vi "Ramsete_Execute_PackTuning_ENG.vi"(5 "B":dbl=2.0, 6 "Heading Tolerance DEG":dbl=0.035, 7 "Zeta":dbl=0.7, 8 "Y Tolerance Ft":dbl=0.051, 9 "X Tolerance Ft":dbl=0.051, 10 "Max Speed Ft/S":dbl, 11 "Track Width Ft":dbl) -> (3 "RAMSETE_EXE_TUNING":T1={"B"=2.0, "Zeta"=0.7, "X Tolerance M"=2.0, "Y Tolerance M"=0.7, "Heading Tolerance RAD"=0.7, "Track Width M"=2.0, "Max Speed M/S"=2.0} {"Max Speed M/S" format="%13.4f"; "Track Width M" format="%13.4f"; "Heading Tolerance RAD" format="%13.4f"; "Y Tolerance M" format="%13.4f"; "X Tolerance M" format="%13.4f"; "Zeta" format="%13.4f"; "B" format="%13.4f"})   [LabVIEW 2019, in "Trajectory_Library.lvlib"]
doc: "Packs tuning parameters for the Ramsete EXE VI (Which is designed for a differential drive robot)\n\nThis verion uses ENG input units (Ft, Degs)"
uses:
  RAMSETE_EXE_TUNING.ctl
  Trajectory_Library.lvlib
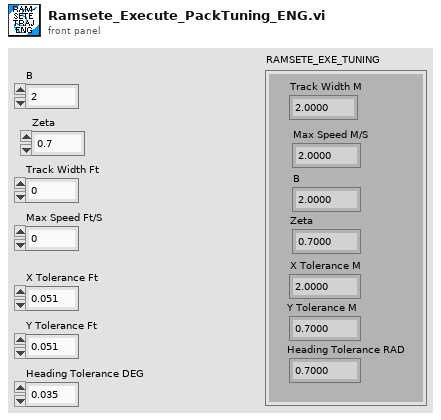
[diagram p1: front panel]
types:
  T1 = typedef "Trajectory_Library.lvlib/RAMSETE_EXE_TUNING.ctl" = cluster{"B":dbl, "Zeta":dbl, "X Tolerance M":dbl, "Y Tolerance M":dbl, "Heading Tolerance RAD":dbl, "Track Width M":dbl, "Max Speed M/S":dbl}
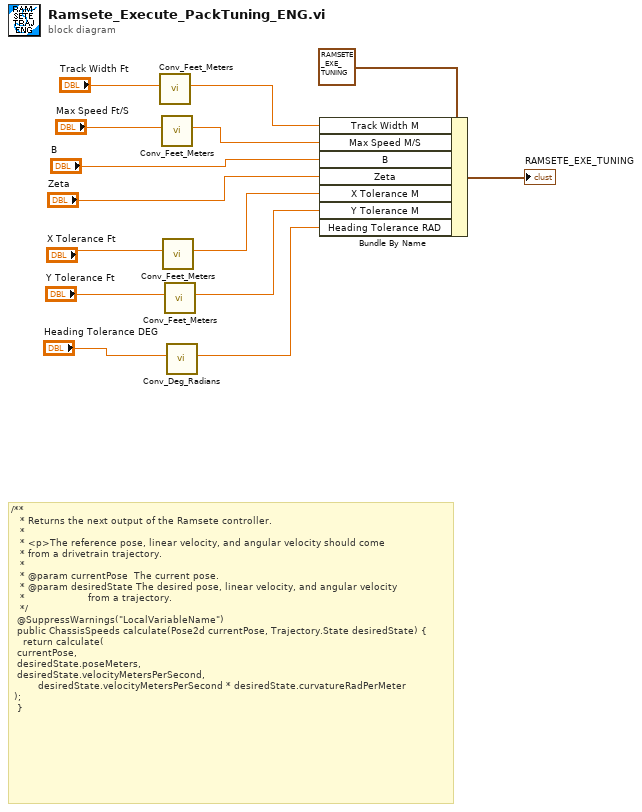
[diagram p0: block diagram]
diagram:
  # "/**\n   * Returns the next output of the Ramsete controller.\n   *\n   * <p>The reference pose, linear velocity, and angular velocity should come\n   * from a drivetrain trajectory.\n   *\n   * @param currentPose  The current pose.\n   * @param desiredState The desired pose, linear velocity, and angular velocity\n   *                     from a trajectory.\n   */\n  @SuppressWarnings(\"LocalVariableName\")\n  public ChassisSpeeds calculate(Pose2d currentPose, Trajectory.State desiredState) {\n    return calculate(\n\t\tcurrentPose, \n\t\tdesiredState.poseMeters, \n\t\tdesiredState.velocityMetersPerSecond,\n        \tdesiredState.velocityMetersPerSecond * desiredState.curvatureRadPerMeter\n\t);\n  }"
  n1 = call "Conv_Feet_Meters.vi"("Feet"="Track Width Ft") -> ("Meters"=w1:dbl)  [unwired: 10 in]
  n2 = call "Conv_Feet_Meters.vi"("Feet"="Max Speed Ft/S") -> ("Meters"=w4:dbl)  [unwired: 10 in]
  n3 = call "Conv_Feet_Meters.vi"("Feet"="X Tolerance Ft") -> ("Meters"=w6:dbl)  [unwired: 10 in]
  n4 = call "Conv_Feet_Meters.vi"("Feet"="Y Tolerance Ft") -> ("Meters"=w8:dbl)  [unwired: 10 in]
  n5 = call "Conv_Deg_Radians.vi"("Degress"="Heading Tolerance DEG") -> ("Radians"=w10:dbl)  [unwired: 10 in]
  n6 = Bundle By Name(cluster=T1 {"B"=2.0, "Zeta"=0.7, "X Tolerance M"=0.051, "Y Tolerance M"=0.051, "Heading Tolerance RAD"=0.035, "Track Width M"=2.0, "Max Speed M/S"=2.0} ("RAMSETE_EXE_TUNING"), "Track Width M"=w1, "Max Speed M/S"=w4, "B"="B", "Zeta"="Zeta", "X Tolerance M"=w6, "Y Tolerance M"=w8, "Heading Tolerance RAD"=w10) -> (→"RAMSETE_EXE_TUNING":T1)
